vi "PID control XYZ R.vi"(0 "x location (um)":dbl, 1 "x polarity":bool, 2 "y polarity":bool, 3 "z polarity":bool, 5 "y location (um)":dbl, 7 "z location (um)":dbl, 9 "measurement time":dbl, 11 "reinitialize? (F)":bool, 12 "XY pos range (um)":cluster{"output high":dbl, "output low":dbl}={"output high"=1000.0, "output low"=-1000.0} {"output low" format="%.2f"; "output high" format="%.2f"}, 13 "z position range (um)":cluster{"output high":dbl, "output low":dbl}={"output high"=100.0, "output low"=-100.0} {"output low" format="%.2f"; "output high" format="%.2f"}, 14 "XY gains":T1={"proportional gain (Kc)"=0.7, "integral time (Ti, sec)"=1.0, "derivative time (Td, sec)"=0.0} {"derivative time (Td, sec)" format="%.3f"; "integral time (Ti, sec)" format="%.3f"; "proportional gain (Kc)" format="%.3f"}, 15 "Z gains":T1={"proportional gain (Kc)"=0.7, "integral time (Ti, sec)"=1.0, "derivative time (Td, sec)"=0.0} {"derivative time (Td, sec)" format="%.3f"; "integral time (Ti, sec)" format="%.3f"; "proportional gain (Kc)" format="%.3f"}) -> (4 "x move (um)":dbl, 6 "y move (um)":dbl, 8 "z move (um)":dbl)   [LabVIEW 2010]
uses:
  <vilib>/addons/control/pid/pid.llb/PID (DBL Array).vi
  <vilib>/addons/control/pid/NI_PID_pid.lvlib
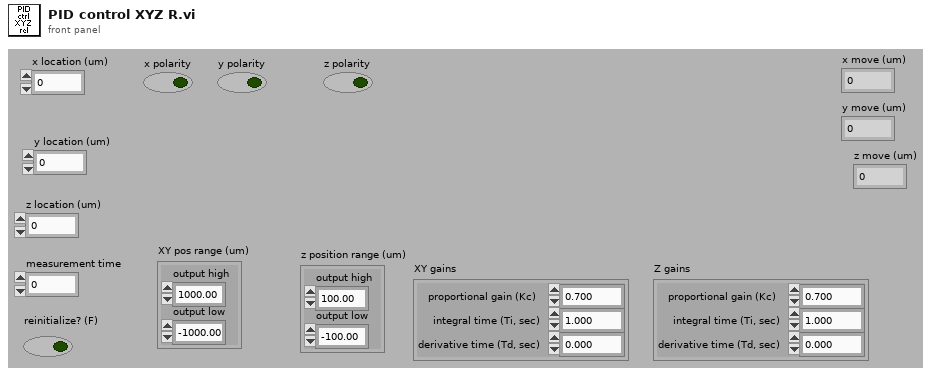
[diagram p1: front panel]
types:
  T1 = cluster{"proportional gain (Kc)":dbl, "integral time (Ti, sec)":dbl, "derivative time (Td, sec)":dbl}
  T2 = cluster{"proportional gain (Kc)":dbl, "integral time (Ti, min)":dbl, "derivative time (Td, min)":dbl}
  T3 = cluster{"proportional gain (Kc)":dbl, "integral time (Ti, min)":dbl, "derivative time (Td, min)":dbl}[]
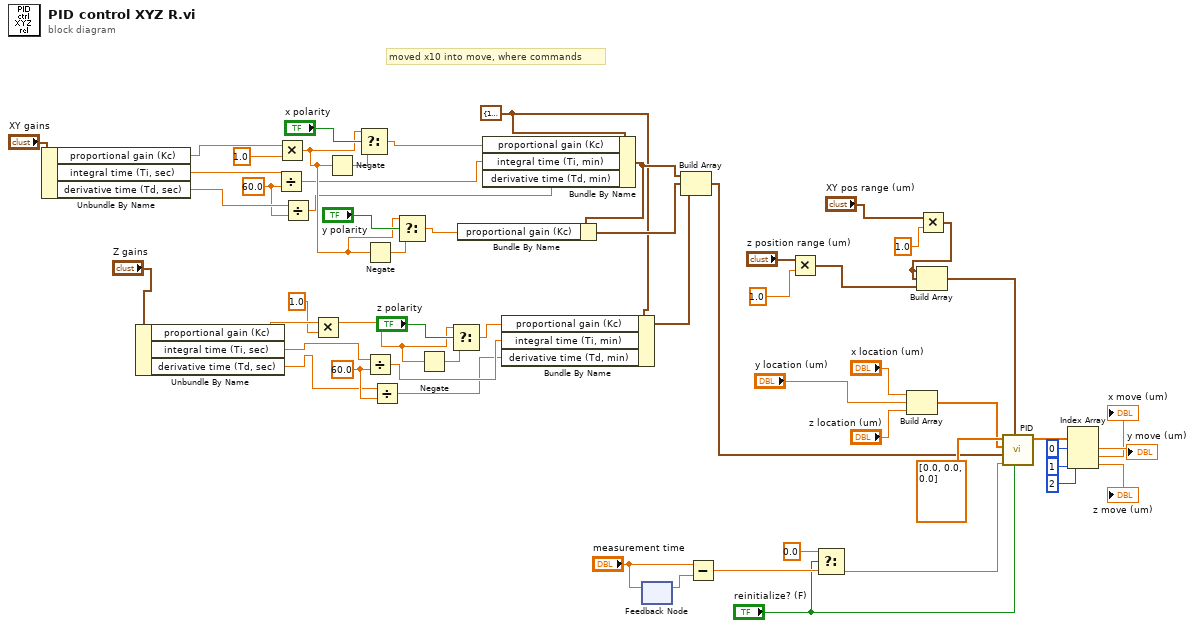
[diagram p0: block diagram]
diagram:
  w11 = 60.0 ("y")
  w50 = 60.0 ("y")
  w12 = T2 {"proportional gain (Kc)"=1.0, "integral time (Ti, min)"=0.01, "derivative time (Td, min)"=0.0} ("Z gains")
  # "moved x10 into move, where commands"
  n1 = Unbundle By Name("XY gains") -> ("proportional gain (Kc)"=w20:dbl, "integral time (Ti, sec)"=w52:dbl, "derivative time (Td, sec)"=w51:dbl)
  n2 = Unbundle By Name("Z gains") -> ("proportional gain (Kc)"=w16:dbl, "integral time (Ti, sec)"=w10:dbl, "derivative time (Td, sec)"=w9:dbl)
  n3 = Divide(x=w52, y=w50) -> (x/y=w43:dbl)
  n4 = Multiply(x=w20, y=1.0) -> (x*y=w45:dbl)
  n5 = Divide(x=w51, y=w50) -> (x/y=w42:dbl)
  n6 = Multiply(x=w16, y=1.0) -> (x*y=w14:dbl)
  n7 = Negate(x=w45) -> (-x=w48:dbl)
  n8 = Select(t=w45, s="x polarity", f=w48) -> (s? t:f=w44:dbl)
  n9 = Negate(x=w45) -> (-x=w46:dbl)
  n10 = Divide(x=w10, y=w11) -> (x/y=w8:dbl)
  n11 = Divide(x=w9, y=w11) -> (x/y=w7:dbl)
  n12 = Select(t=w45, s="y polarity", f=w46) -> (s? t:f=w41:dbl)
  n13 = Negate(x=w14) -> (-x=w17:dbl)
  n14 = Select(t=w14, s="z polarity", f=w17) -> (s? t:f=w15:dbl)
  n15 = Bundle By Name(cluster=w12, "proportional gain (Kc)"=w44, "integral time (Ti, min)"=w43, "derivative time (Td, min)"=w42) -> (w40:T2)
  n16 = Bundle By Name(cluster=w40, "proportional gain (Kc)"=w41) -> (w39:T2)
  n17 = Bundle By Name(cluster=w12, "proportional gain (Kc)"=w15, "integral time (Ti, min)"=w8, "derivative time (Td, min)"=w7) -> (w37:T2)
  n18 = feedback-in #1("measurement time") -> ()
  n19 = feedback #1() -> (w55:dbl)  [unwired: 1 in]
  n20 = Build Array(w40, w39, w37) -> (w36:T3)
  n21 = Subtract(x="measurement time", y=w55) -> (x-y=w54:dbl)
  n22 = Multiply(x="z position range (um)", y=1.0 ("measurement time")) -> (x*y=w30:cluster{"output high":dbl, "output low":dbl})
  n23 = Select(t=0.0, s="reinitialize? (F)", f=w54) -> (s? t:f=w3:dbl)
  n24 = Build Array("x location (um)", "y location (um)", "z location (um)") -> (w29:dbl[])
  n25 = Multiply(x="XY pos range (um)", y=1.0 ("measurement time")) -> (x*y=w4:cluster{"output high":dbl, "output low":dbl})
  n26 = Build Array(w4, w4, w30) -> (w28:cluster{"output high":dbl, "output low":dbl}[])
  n27 = call-poly <vilib>:"PID.vi"("reinitialize? (F)"="reinitialize? (F)", "output range"=w28, "dt (s)"=w3, "PID gains"=w36, "process variable"=w29, "setpoint"=dbl[] [0.0, 0.0, 0.0]) -> ("output"=w27:dbl[])  [unwired: 4 in, 1 out]
  n28 = Index Array(array=w27, index #1=0 ("index"), index #2=1 ("index"), index #3=2 ("index")) -> (element #1=→"y move (um)":dbl, element #2=→"x move (um)":dbl, element #3=→"z move (um)":dbl)
